vi "IP端口 合并 网络地址字符串.vi"(6 "分隔符(:)":string=":", 11 "IP端口":cluster{"IP":string, "Port":u16}) -> (3 "IP端口字符串":string)   [LabVIEW 2017]
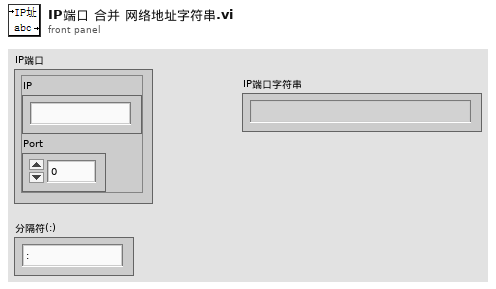
[diagram p1: front panel]
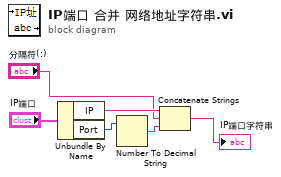
[diagram p0: block diagram]
diagram:
  n1 = Unbundle By Name("IP端口") -> ("IP"=w4:string, "Port"=w5:u16)
  n2 = Number To Decimal String(number=w5) -> (decimal integer string=w2:string)  [unwired: 1 in]
  n3 = Concatenate Strings(w4, "分隔符(:)", w2) -> (→"IP端口字符串":string)
